vi "retract.vi"(8 "error in (no error)":errorcluster, 11 "Input":string="34,45,89") -> (0 "error out":errorcluster, 3 "Output":string)   [LabVIEW 2014]
uses:
  <userlib>/Nanonis Prog Interface V5/Nanonis Prog Interface.lvlib
panel:
  out "steps":i32
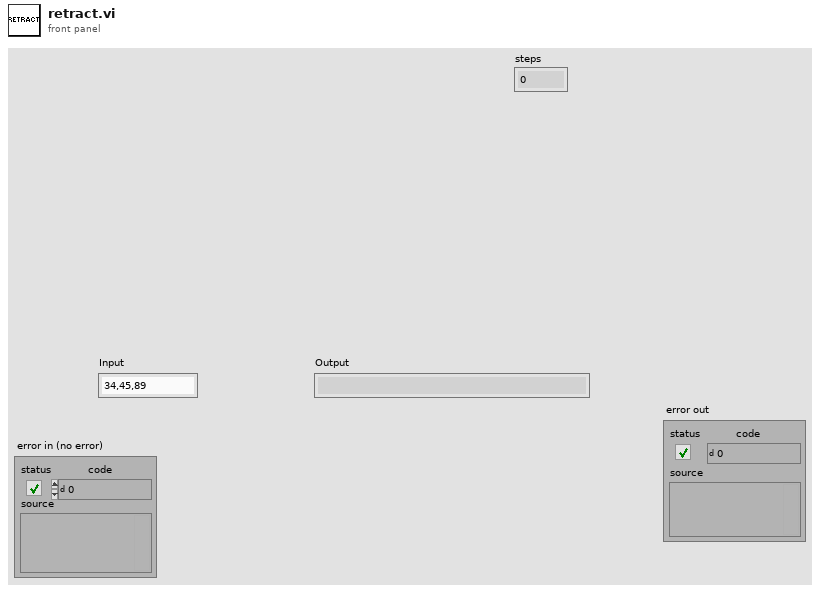
[diagram p1: front panel]
types:
  T1 = enum8{"Group 1", "Group 2", "Group 3", "Group 4", "Group 5", "Group 6"}
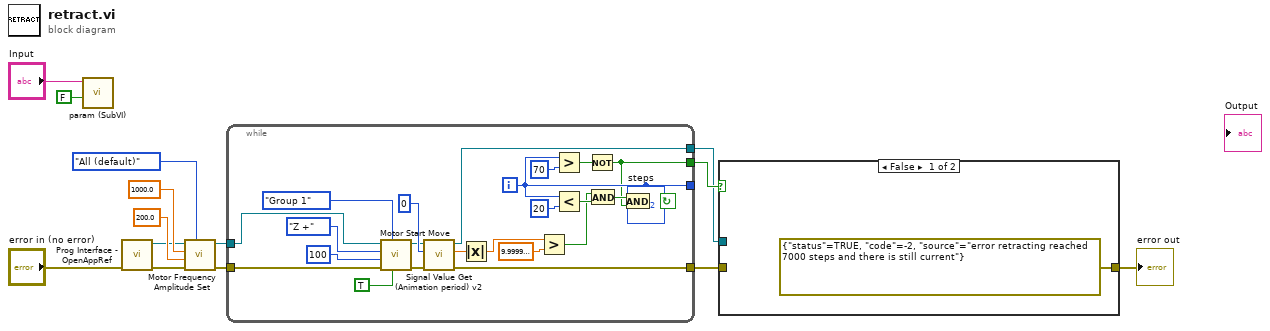
[diagram p0: block diagram]
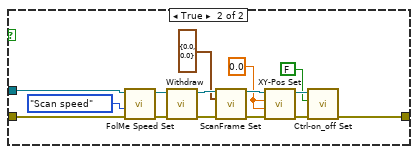
[diagram p2: hidden frame]
diagram:
  n1 = call <userlib>:"param (SubVI).vi"("Numeric"=FALSE, "Input"="Input") -> ()  [unwired: 7 in, 3 out]
  n2 = call <userlib>:"Prog Interface - OpenAppRef.vi"("Error in (no error)"="error in (no error)") -> ("Error out"=w2:errorcluster, "Application reference"=w3:refnum<vi>)  [unwired: 5 in]
  n3 = call <userlib>:"Motor Frequency Amplitude Set.vi"("Axis (All)"=enum16{"All (default)", "X", "Y", "Z"}."All (default)", "Error in (no error)"=w2, "Amplitude (V) (NaN=no change)"=sgl 200.0, "Frequency (Hz) (NaN=no change)"=sgl 1000.0, "Application ref in"=w3) -> ("Error out"=w7:errorcluster, "Application ref out"=w8:refnum<vi>)  [unwired: 5 in]
  n4 = while {
    tunnel: [w27] -> w5
    tunnel: [w26] -> w4
    tunnel: w8 -> [w25]
    tunnel: w7 -> [w24]
    tunnel: [w19] -> _
    tunnel: [w15] -> w6
    i -> [w19]
    stop <- w16 continue-if-true
    n5 = call <userlib>:"Motor Start Move.vi"("Wait until finished? (F)"=TRUE, "Group"=T1."Group 1", "Error in (no error)"=w24, "Number of steps"=u16 100, "Direction"=enum16{"X +", "X -", "Y +", "Y -", "Z +", "Z -"}."Z +", "Application ref in"=w25) -> ("Error out"=w20:errorcluster, "Application ref out"=w21:refnum<vi>)  [unwired: 3 in]
    n6 = call <userlib>:"Signal Value Get (Animation period) v2.vi"("error in (no error)"=w20, "Signal index (0-79)"=i8 0, "Application ref in"=w21) -> ("error out"=w26:errorcluster, "Signal value"=w33:sgl, "Application ref out"=w27:refnum<vi>)  [unwired: 5 in]
    n7 = Absolute Value(x=w33) -> (abs(x)=w31:sgl)
    n8 = Greater?(x=w31, y=sgl 1e-11) -> (0:w23:bool)
    n9 = Greater?(x=w19, y=70) -> (0:w17:bool)
    n10 = Less?(x=w19, y=20) -> (x < y?=w28:bool)
    n11 = Not(x=w17) -> (.not. x?=w15:bool)
    n12 = And(x=w23, y=w28) -> (x .and. y?=w29:bool)
    n13 = And(x=w29, y=w15) -> (x .and. y?=w16:bool)
    "steps" <- w19
  }
  n14 = case shown="False" w6 {
    tunnel: w5 -> [_ w41]
    tunnel: w4 -> [_ w40]
    tunnel: [errorcluster {"status"=TRUE, "code"=-2, "source"="error retracting reached 7000 steps and there is still current"} ("error out") w39] -> w1
    frame False {
    }
    frame True {
      w48 = sgl 0.0 ("X (m)")
      n15 = call <userlib>:"FolMe Speed Set.vi"("error in (no error)"=w40, "Speed Setting (Custom)"=enum32{"Scan speed", "Custom speed"}."Scan speed", "Application ref in"=w41) -> ("error out"=w45:errorcluster, "Application ref out"=w46:refnum<vi>)  [unwired: 5 in]
      n16 = call <userlib>:"Withdraw.vi"("Error in (no error)"=w45, "Application ref in"=w46) -> ("Error out"=w52:errorcluster, "Application ref out"=w53:refnum<vi>)  [unwired: 8 in]
      n17 = call <userlib>:"ScanFrame Set.vi"("Application ref in"=w53, "Center coordinates (m)"=cluster{"Xc":sgl, "Yc":sgl} {"Xc"=0.0, "Yc"=0.0}, "error in (no error)"=w52) -> ("Application ref out"=w49:refnum<vi>, "error out"=w50:errorcluster)  [unwired: 11 in]
      n18 = call <userlib>:"XY-Pos Set.vi"("error in (no error)"=w50, "Y (m)"=w48, "X (m)"=w48, "Application ref in"=w49) -> ("error out"=w43:errorcluster, "Application ref out"=w44:refnum<vi>)  [unwired: 4 in]
      n19 = call <userlib>:"Ctrl-on_off Set.vi"("error in (no error)"=w43, "Z Controller ON/OFF"=FALSE, "Application ref in"=w44) -> ("error out"=w39:errorcluster)  [unwired: 7 in, 1 out]
    }
  }
  "error out" <- w1
